vi "Pre Launch Init.vi"(11 "Tracer-P in":refnum<class "Tracer-P.lvclass">) -> (0 "error out":errorcluster, 3 "Tracer-P out":refnum<class "Tracer-P.lvclass">)   [LabVIEW 2013, in "Tracer-P.lvclass"]
doc: "(<B>Filename</B>: Actor Framework.lvlib:Actor.lvclass:Pre Launch Init.vi)\n\nDefines behavior that occurs after the Launch Actor method is invoked but before the actor's Actor Core method begins running.\n\nThe Pre Launch Init method is guaranteed to finish before the Launch Actor method returns to its caller and before the actor itself receives any messages. Any references that the Pre Launch Init method obtains are guaranteed to have the same lifetime as the actor itself. Any errors that the Pre Launch Init method returns will abort the launch.\n\nBy default, this method does nothing. A descendant class may override it to define behavior."
uses:
  Tracer-P.lvclass
  Tracer-P.lvclass/Tracer-P.ctl
  Logical Systems/Tracer/Tracer.lvclass
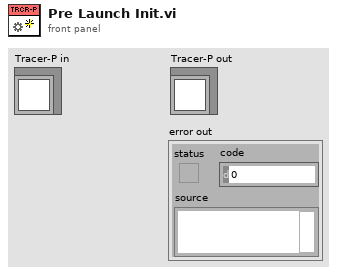
[diagram p1: front panel]
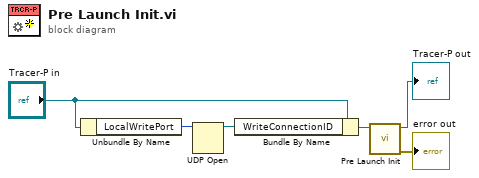
[diagram p0: block diagram]
diagram:
  n1 = Unbundle By Name("Tracer-P in") -> ("LocalWritePort"=w3:u16)
  n2 = UDP Open(11:w3) -> (port=w1:refnum<k16>)  [unwired: 4 in, 2 out]
  n3 = Bundle By Name(cluster="Tracer-P in", "WriteConnectionID"=w1) -> (w2:refnum<class "Tracer-P.lvclass">)
  n4 = call-parent "Pre Launch Init.vi"("Actor in"=w2) -> ("error out"=→"error out":errorcluster, "Actor out"=→"Tracer-P out":refnum<class "Tracer-P.lvclass">)  [unwired: 9 in]
